vi "RichToFlatnidaqmx_grpc_SetChanAttributeStringResponse.vi"(5 "OutputClusterType":T1, 11 "InputCluster":T2) -> (3 "OutputCluster":T1)   [LabVIEW 2021, in "NI DAQmx_server.lvlib"]
uses:
  NI DAQmx_server.lvlib
  nidaqmx_grpc_SetChanAttributeStringResponse.ctl
  nidaqmx_grpc_SetChanAttributeStringResponse_Flat.ctl
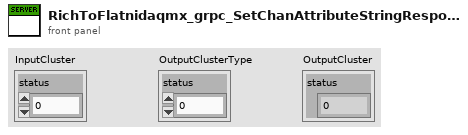
[diagram p1: front panel]
types:
  T1 = typedef "NI DAQmx_server.lvlib/nidaqmx_grpc_SetChanAttributeStringResponse_Flat.ctl" = cluster{"status":i32}
  T2 = typedef "NI DAQmx_server.lvlib/nidaqmx_grpc_SetChanAttributeStringResponse.ctl" = cluster{"status":i32}
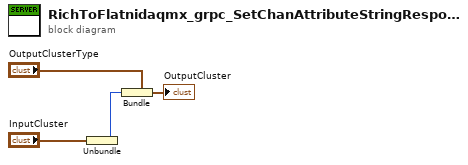
[diagram p0: block diagram]
diagram:
  n1 = Unbundle "Unbundle"("InputCluster") -> ("status"=w1:i32)
  n2 = Bundle "Bundle"(cluster="OutputClusterType", "status"=w1) -> (→"OutputCluster":T1)
